vi "Save_to_Project.vi"(8 "error in (no error)":errorcluster, 9 "index in":string, 10 "buildObject":T2, 11 "IB_RegDest in":refnum<class "IB_RegDest.lvclass">) -> (0 "error out":errorcluster, 1 "index out":string, 2 "buildObject out":T2, 3 "IB_RegDest out":refnum<class "IB_RegDest.lvclass">, 5 "saved?":bool)   [LabVIEW 2020, in "IB_RegDest.lvclass"]
uses:
  <vilib>/AppBuilder/IB_Classes/RegDest/IB_RegDest.lvclass
  <vilib>/AppBuilder/IB_Classes/RegDest/IB_RegDest.lvclass/IB_RegDest.ctl
  <vilib>/AppBuilder/IB_RW_Project/IB_RW_Project_PropBag_Action.ctl
  <resource>/Framework/Providers/API/ItemRef.ctl
  <vilib>/AppBuilder/IB_RW_Project/IB_RW_Project_RegDest_Data.ctl
panel:
  in  "data":T1
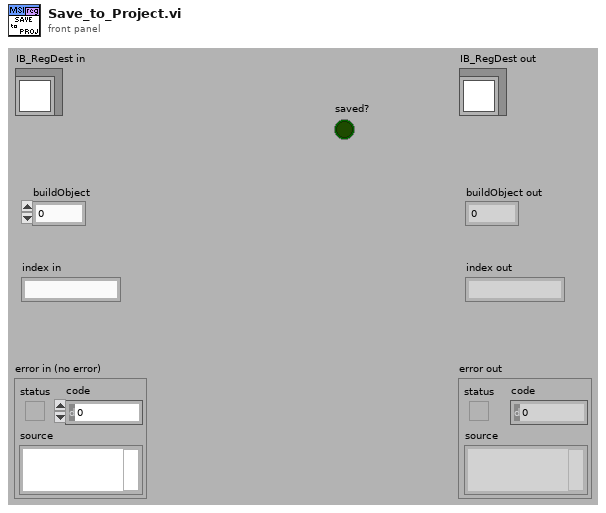
[diagram p1: front panel]
types:
  T1 = typedef "IB_RW_Project_RegDest_Data.ctl" = cluster{"parentTag":string, "dirTag":string, "dirName":string, "unlock":bool}
  T2 = typedef "ItemRef.ctl" = u64
  T3 = typedef "IB_RW_Project_PropBag_Action.ctl" = enum16{"read", "write", "clear", "readPrevious", "writePrevious", "clearPrevious"}
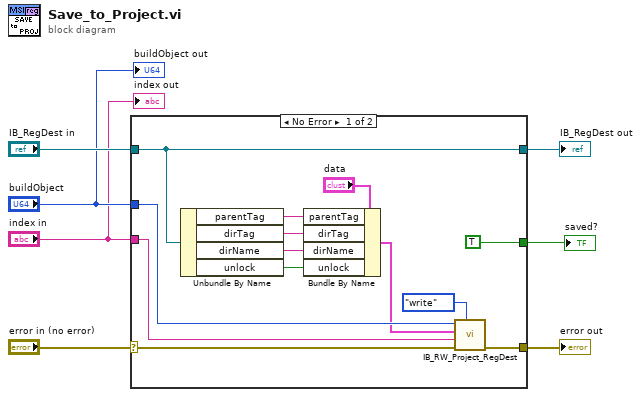
[diagram p0: block diagram]
diagram:
  n1 = case shown="No Error" "error in (no error)" {
    selector: "error in (no error)" -> [w12 w22]
    tunnel: [w11 w22] -> w6
    tunnel: [w20 w21] -> w4
    tunnel: "IB_RegDest in" -> [w20 w21]
    tunnel: "buildObject" -> [w10 _]
    tunnel: "index in" -> [w13 _]
    tunnel: [TRUE _] -> w1
    frame No Error {
      n2 = Unbundle By Name(w20) -> ("parentTag"=w18:string, "dirTag"=w17:string, "dirName"=w16:string, "unlock"=w15:bool)
      n3 = Bundle By Name(cluster="data", "parentTag"=w18, "dirTag"=w17, "dirName"=w16, "unlock"=w15) -> (w9:T1)
      n4 = call <vilib>:"IB_RW_Project_RegDest.vi"("action"=IB_RW_Project_PropBag_Action."write", "error in (no error)"=w12, "index in"=w13, "RegDest"=w9, "buildObject"=w10) -> ("error out"=w11:errorcluster)  [unwired: 3 in, 3 out]
    }
    frame Error {
    }
  }
  "error out" <- w6
  "IB_RegDest out" <- w4
  "saved?" <- w1
  "buildObject out" <- "buildObject"
  "index out" <- "index in"
